vi "Application Demo.vi"() -> ()   [LabVIEW 2024]
uses:
  Libraries/UIs Handler/UIs/Select UI.ctl
  Libraries/UIs Handler/UIs Handler.lvlib
panel:
  in  "Close":bool
  in  "Select UI":string(combo)
  out "Status":string
  out "Error out":errorcluster
  out "Module Was Already Running?":bool
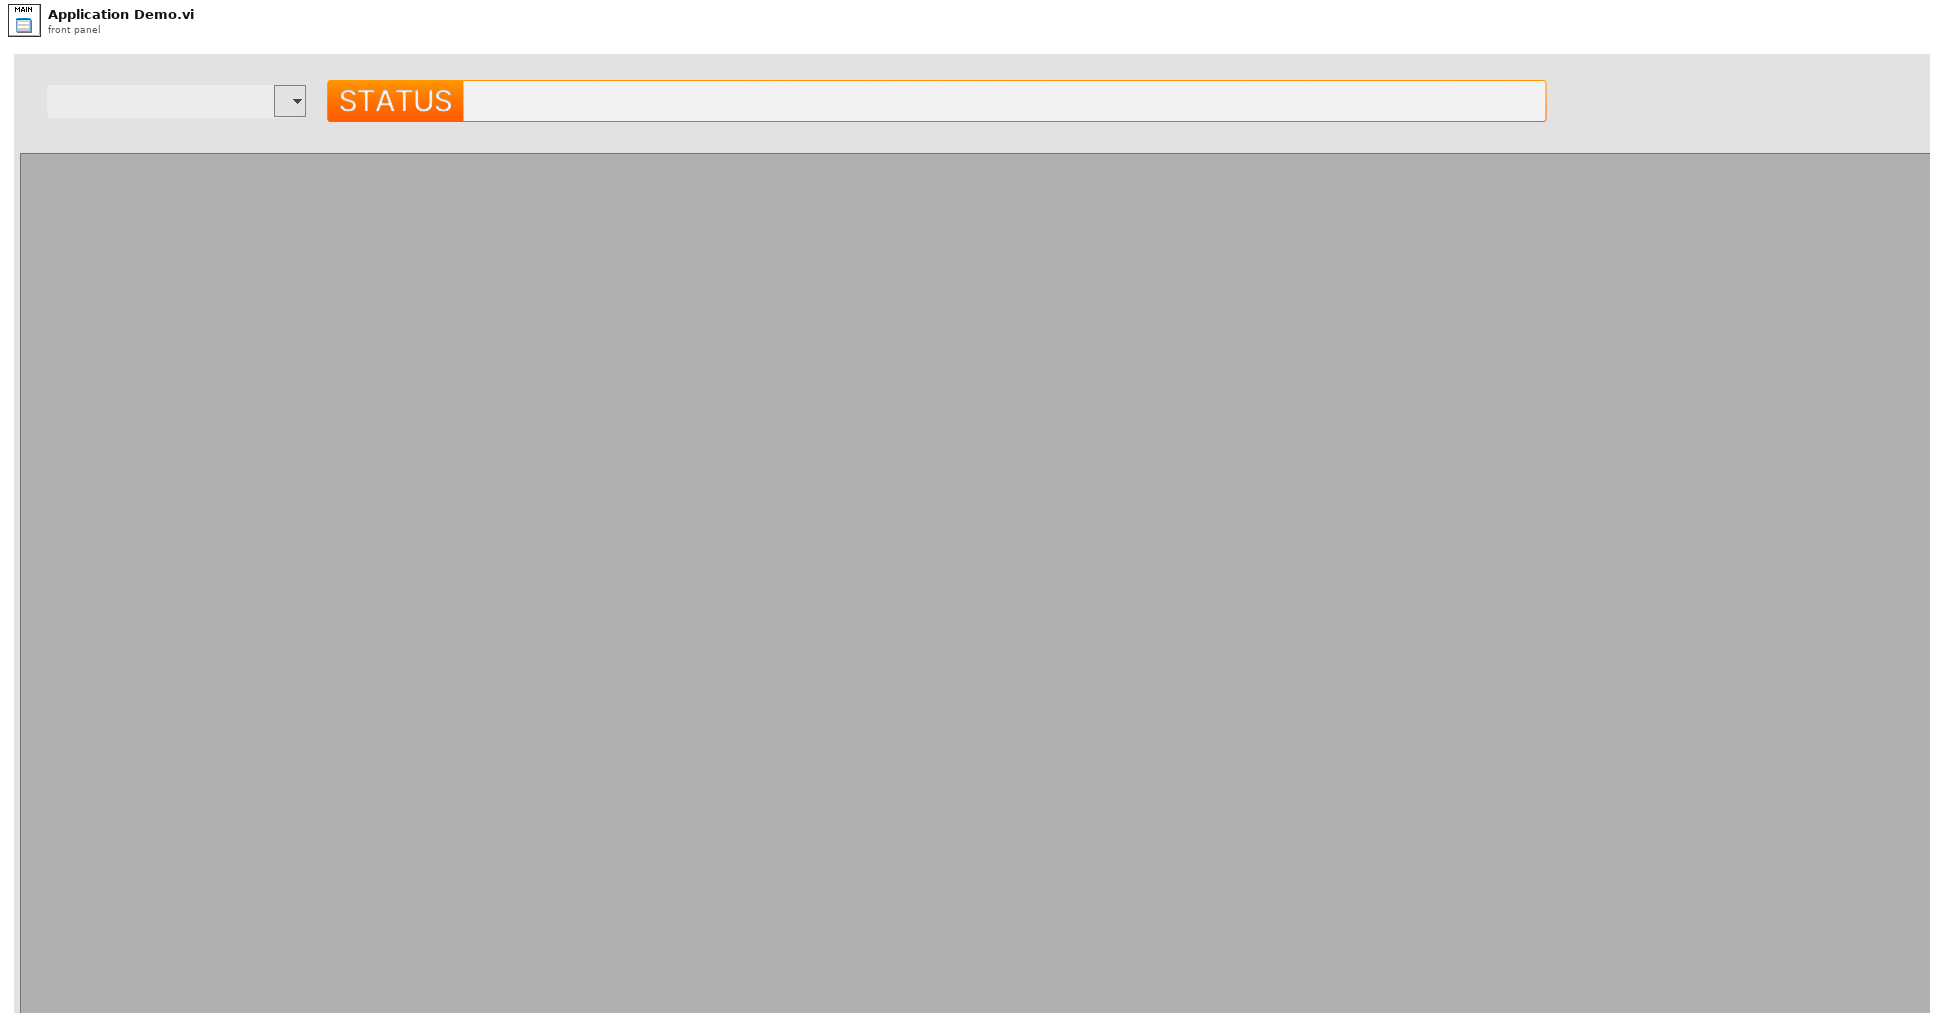
[diagram p1: front panel]
types:
  T1 = typedef "UIs Handler.lvlib/Broadcast Events--cluster.ctl" = cluster{"Module Did Init":refnum<user-event>, "Status Updated":refnum<user-event>, "Error Reported":refnum<user-event>, "Module Did Stop":refnum<user-event>, "Update Module Execution Status":refnum<user-event>, "Update Data":refnum<user-event>}
  T2 = typedef "UIs Handler.lvlib/Select UI.ctl" = enum16{"Dashboard", "Meta Tabs"}
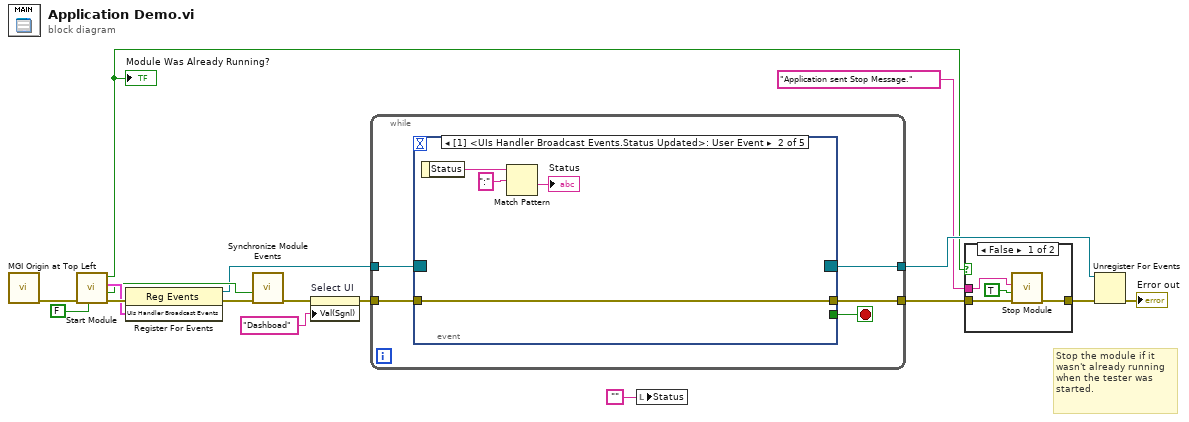
[diagram p0: block diagram]
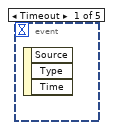
[diagram p3: hidden frame]
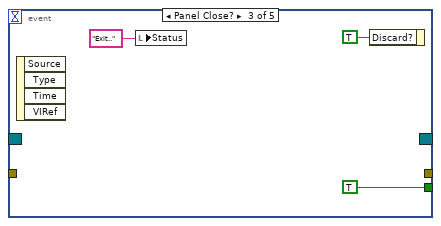
[diagram p4: hidden frame]
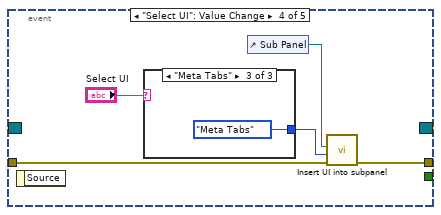
[diagram p5: hidden frame]
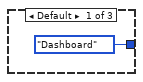
[diagram p6: hidden frame]
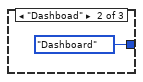
[diagram p7: hidden frame]
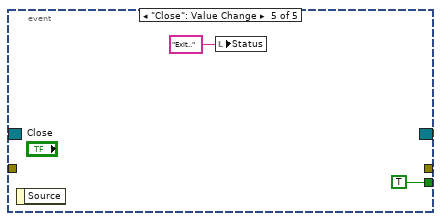
[diagram p8: hidden frame]
diagram:
  # "Stop the module if it wasn't already running when the tester was started."
  n1 = call <userlib>:"MGI Origin at Top Left.vi"() -> ("Error Out"=w11:errorcluster)  [unwired: 9 in, 1 out]
  n2 = call "Start Module.vi"("Show Main VI Diagram on Init (F)"=FALSE, "error in"=w11) -> ("error out"=w16:errorcluster, "Wait for Event Sync?"=w13:bool, "UIs Handler Broadcast Events"=w15:T1, "Module Was Already Running?"=w5:bool)  [unwired: 5 in, 1 out]
  "Module Was Already Running?" <- w5
  n3 = register-events(error in=w16, w15) -> (reference out=w12:refnum<event-registration>, error out=w17:errorcluster)  [unwired: 1 in]
  n4 = call "Synchronize Module Events.vi"("error in"=w17, "Wait for Event Sync?"=w13) -> ("error out"=w3:errorcluster)  [unwired: 9 in]
  n5 = property on="Select UI" class="CmbBox"(error in=w3, "Val(Sgnl)"="Dashboad" ("Value (Signaling)")) -> (error out=w2:errorcluster)  [unwired: 1 in, 1 out]
  n6 = while {
    tunnel: w2 -> [w19]
    tunnel: w12 -> [w22]
    tunnel: [w20] -> w8
    tunnel: [w18] -> w7
    stop <- w21 stop-if-true
    n7 = event shown="[1] <UIs Handler Broadcast Events.Status Updated>: User Event" {
      selector: w22 -> [_ _ _ _ _]
      dyn-events: [_ _ _ _ _] -> w20
      timeout: _ -> [_ _ _ _ _]
      tunnel: [_ _ TRUE _ TRUE] -> w21
      tunnel: [_ w23 _ w31 _] -> w18
      tunnel: w19 -> [_ w23 _ w30 _]
      event Timeout {
        n8 = event-data() -> ()  [unwired: 1 in, 3 out]
      }
      event User Event {
        n9 = event-data() -> ("Status"=w26:string)  [unwired: 1 in]
        n10 = Match Pattern(string=w26, regular expression=":") -> (after substring=→"Status":string)  [unwired: 1 in, 3 out]
      }
      event Panel Close? {
        n11 = event-data() -> ()  [unwired: 1 in, 4 out]
        n12 = local write "Status"("Exit.." ("Status")) -> ()
        n13 = event-data("Discard?"=TRUE) -> ()  [unwired: 1 in, 1 out]
      }
      event "Select UI": Value Change {
        n14 = event-data() -> ()  [unwired: 1 in, 1 out]
        n15 = case shown="\"Meta Tabs\"" "Select UI" {
          tunnel: [Select_UI."Dashboard" ("Select UI") Select_UI."Dashboard" ("Select UI") Select_UI."Meta Tabs" ("Select UI")] -> w32
          frame Default {
          }
          frame "Dashboad" {
          }
          frame "Meta Tabs" {
          }
        }
        n16 = control-ref of="Sub Panel"() -> (w34:refnum<vi>)
        n17 = call "Insert UI into subpanel.vi"("error in"=w30, "Select UI"=w32, "Subpanel"=w34) -> ("error out"=w31:errorcluster)  [unwired: 8 in]
      }
      event "Close": Value Change {
        n18 = event-data() -> ()  [unwired: 1 in, 1 out]
        n19 = local write "Status"("Exit.." ("Status")) -> ()
      }
    }
  }
  n20 = local write "Status"("") -> ()
  n21 = case shown="False" w5 {
    tunnel: [w43 w44] -> w9
    tunnel: "Application sent Stop Message." ("Origin") -> [w42 _]
    tunnel: w7 -> [w40 w44]
    frame False {
      n22 = call "Stop Module.vi"("error in"=w40, "Wait for Module to Stop? (F)"=TRUE ("Wait for Module to stop?"), "Origin"=w42) -> ("error out"=w43:errorcluster)  [unwired: 8 in]
    }
    frame True {
    }
  }
  n23 = Unregister For Events(event registration refnum=w8, error in=w9) -> (error out=→"Error out":errorcluster)
